vi "datasourceConfigs.from_json.vi"(8 "error in":errorcluster, 10 "json":string) -> (0 "error out":errorcluster, 2 "datasourceConfigs":T1[](array[typedef]))   [LabVIEW 2020, in "type.lvclass"]
uses:
  type.lvclass
  datasourceConfig.ctl
  7f84b30d-55bd-48c8-8d63-fe38355a9436.vi
  <vilib>/JDP Science/JSONtext/JSON text to Variant.vi
  <vilib>/JDP Science/JSONtext/LVClass Serializer/JSONtext LVClass Serializer.lvclass
  <vilib>/JDP Science/JSONtext/JSONtext.lvlib
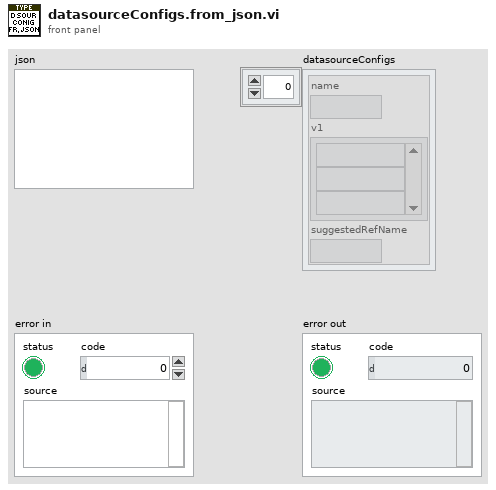
[diagram p1: front panel]
types:
  T1 = typedef "type.lvclass/datasourceConfig.ctl" = cluster{"name":string, "v1":string[], "suggestedRefName":string}
  T2 = cluster{"tags":cluster{"type":string, "v1":string[]}, "suggestedRefName":string}
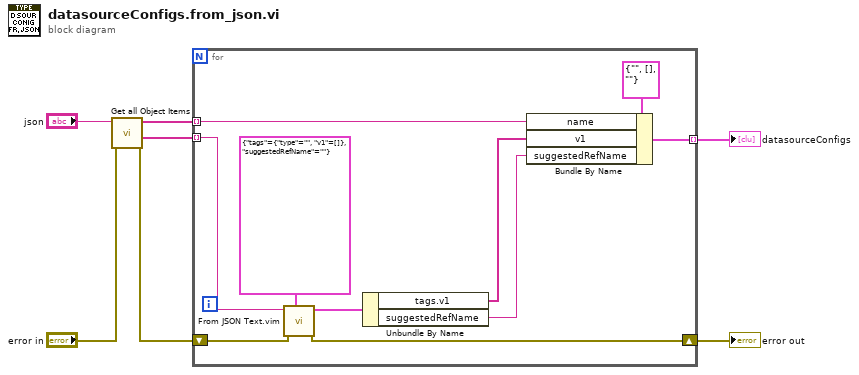
[diagram p0: block diagram]
diagram:
  n1 = call <vilib>:"Get all Object Items.vi"("error in (no error)"="error in", "JSON"="json") -> ("error out"=w3:errorcluster, "<JSON>"=w4:string[], "Item Names"=w5:string[])  [unwired: 6 in, 1 out]
  n2 = for {
    tunnel: w5 -> [w14] mode=indexing
    tunnel: w4 -> [w16] mode=indexing
    shift-right: [w9] -> w1
    shift-left: w3 -> [w10]
    tunnel: [w8] -> w2 mode=indexing
    n3 = call "From JSON Text.vim"("Data Type and Default Value"=T2 {"tags"={"type"="", "v1"=[]}, "suggestedRefName"=""}, "error in (no error)"=w10, "JSON"=w16) -> ("error out"=w9:errorcluster, "Data out"=w13:T2)  [unwired: 7 in]
    n4 = Unbundle By Name(w13) -> ("tags.v1"=w12:string[], "suggestedRefName"=w11:string)
    n5 = Bundle By Name(cluster=T1 {"name"="", "v1"=[], "suggestedRefName"=""} ("datasource config"), "name"=w14, "v1"=w12, "suggestedRefName"=w11) -> (w8:T1)
  }
  "datasourceConfigs" <- w2
  "error out" <- w1
